vi "Set TDMS File Group Properties.vi"(8 "error in (no error)":errorcluster, 10 "Log File Properties":T1, 11 "Refnum in":refnum<k34>) -> (0 "error out":errorcluster, 3 "Refnum out":refnum<k34>)   [LabVIEW 2019, in "Telemetry Engine.lvlib"]
uses:
  Telemetry Engine.lvlib
  Types/Log File Properties.ctl
  Shared/Constants.vi
  Shared/Telemetry Shared.lvlib
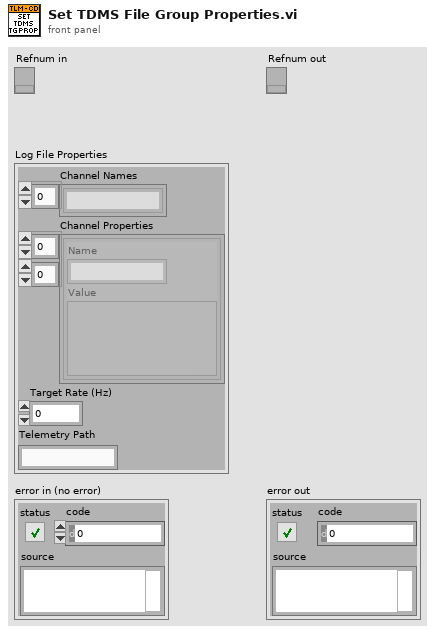
[diagram p1: front panel]
types:
  T1 = typedef "Telemetry Engine.lvlib/Log File Properties.ctl" = cluster{"Channel Names":string[], "Channel Properties":cluster{"Name":string, "Value":variant}[][], "Target Rate (Hz)":dbl, "Telemetry Path":string}
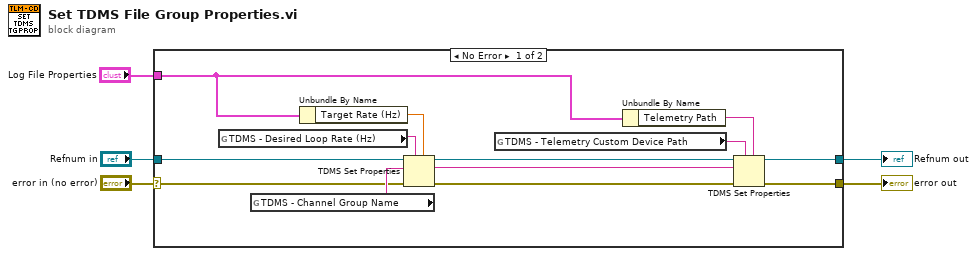
[diagram p0: block diagram]
diagram:
  n1 = case shown="No Error" "error in (no error)" {
    selector: "error in (no error)" -> [w15 w20]
    tunnel: "Log File Properties" -> [w8 _]
    tunnel: "Refnum in" -> [w17 w19]
    tunnel: [w10 w19] -> w3
    tunnel: [w11 w20] -> w2
    frame No Error {
      n2 = global read "Constants.vi" "TDMS - Desired Loop Rate (Hz)"() -> (w14:string)
      n3 = global read "Constants.vi" "TDMS - Channel Group Name"() -> (w16:string)
      n4 = Unbundle By Name(w8) -> ("Target Rate (Hz)"=w18:dbl)
      n5 = TDMS Set Properties(5:w18, 7:w14, 8:w15, 10:w16, 11:w17) -> (0:w12:errorcluster, 2:w9:string, 3:w13:refnum<k34>)  [unwired: 1 in, 1 out]
      n6 = global read "Constants.vi" "TDMS - Telemetry Custom Device Path"() -> (w6:string)
      n7 = Unbundle By Name(w8) -> ("Telemetry Path"=w7:string)
      n8 = TDMS Set Properties(5:w7, 7:w6, 8:w12, 10:w9, 11:w13) -> (0:w11:errorcluster, 3:w10:refnum<k34>)  [unwired: 1 in, 2 out]
    }
    frame Error {
    }
  }
  "Refnum out" <- w3
  "error out" <- w2
